vi "ExampleReader.vi"() -> ()   [LabVIEW 2011]
uses:
  Reader/readType.ctl
  2-Think/2 Typedefs/eStopCommand.ctl
  Reader/NetworkStreamReader.lvclass
panel:
  out "data 2":i32
  out "element 2":variant
  in  "Read Type":T1=enum."Most current"
  in  "Loop delay (ms)":u32
  out "element":variant
  out "data":i32
  # "Note: writer is running at 50 ms"
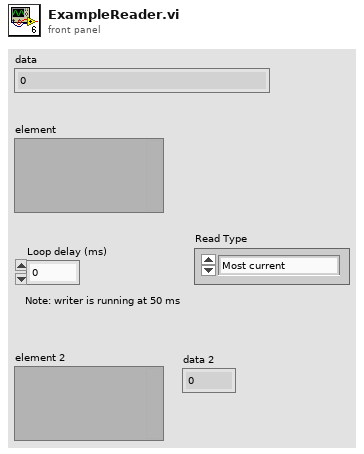
[diagram p1: front panel]
types:
  T1 = typedef "NetworkStreamReader.lvclass/readType.ctl" = enum16{"Next in buffer", "Most current"}
  T2 = typedef "eStopCommand.ctl" = enum16{"Reset E-Stop", "Get E-Stop", "Set E-Stop"}
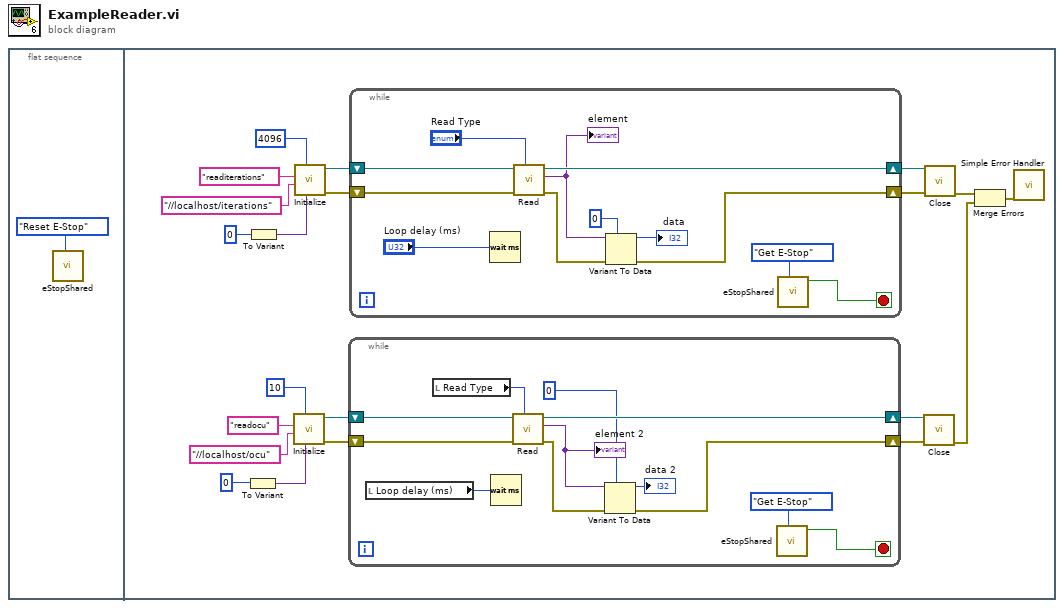
[diagram p0: block diagram]
diagram:
  n1 = flat-sequence {
    frame #0 {
      n2 = call "eStopShared.vi"("Command"=eStopCommand."Reset E-Stop") -> ()  [unwired: 9 in, 2 out]
    }
    frame #1 {
      n3 = To Variant(anything=0) -> (Variant=w13:variant)
      n4 = To Variant(anything=0) -> (Variant=w14:variant)
      n5 = call "Initialize.vi"("Default return"=w13, "writer buffer size"=10, "writer url"="//localhost/ocu", "reader name"="readocu") -> ("error out"=w6:errorcluster, "NetworkStreamWriter out"=w10:refnum<class "NetworkStreamReader.lvclass">)  [unwired: 6 in]
      n6 = call "Initialize.vi"("Default return"=w14, "writer buffer size"=4096, "writer url"="//localhost/iterations", "reader name"="readiterations") -> ("error out"=w22:errorcluster, "NetworkStreamWriter out"=w18:refnum<class "NetworkStreamReader.lvclass">)  [unwired: 6 in]
      n7 = while {
        shift-right: [w32] -> w12
        shift-left: w10 -> [w34]
        shift-right: [w23] -> w11
        shift-left: w6 -> [w33]
        stop <- w29 stop-if-true
        n8 = local read "Loop delay (ms)"() -> (w27:u32)
        n9 = local read "Read Type"() -> (w28:T1)
        n10 = Wait (ms)(milliseconds to wait=w27) -> ()  [unwired: 1 out]
        n11 = call "Read.vi"("Read Type"=w28, "error in (no error)"=w33, "NetworkStreamReader in"=w34) -> ("error out"=w24:errorcluster, "element"=w31:variant, "NetworkStreamReader out"=w32:refnum<class "NetworkStreamReader.lvclass">)  [unwired: 6 in]
        "element 2" <- w31
        n12 = Variant To Data(error in=w24, type=0, Variant=w31) -> (data=→"data 2":i32, error out=w23:errorcluster)
        n13 = call "eStopShared.vi"("Command"=eStopCommand."Get E-Stop") -> ("E-Stop Out"=w29:bool)  [unwired: 9 in, 1 out]
      }
      n14 = while {
        shift-right: [w44] -> w16
        shift-left: w18 -> [w46]
        shift-right: [w35] -> w17
        shift-left: w22 -> [w45]
        stop <- w37 stop-if-true
        n15 = Wait (ms)(milliseconds to wait="Loop delay (ms)") -> ()  [unwired: 1 out]
        n16 = call "Read.vi"("Read Type"="Read Type", "error in (no error)"=w45, "NetworkStreamReader in"=w46) -> ("error out"=w36:errorcluster, "element"=w43:variant, "NetworkStreamReader out"=w44:refnum<class "NetworkStreamReader.lvclass">)  [unwired: 6 in]
        "element" <- w43
        n17 = Variant To Data(error in=w36, type=0, Variant=w43) -> (data=→"data":i32, error out=w35:errorcluster)
        n18 = call "eStopShared.vi"("Command"=eStopCommand."Get E-Stop") -> ("E-Stop Out"=w37:bool)  [unwired: 9 in, 1 out]
      }
      n19 = call "Close.vi"("error in (no error)"=w11, "NetworkStreamReader in"=w12) -> ("error out"=w4:errorcluster)  [unwired: 8 in, 1 out]
      n20 = call "Close.vi"("error in (no error)"=w17, "NetworkStreamReader in"=w16) -> ("error out"=w5:errorcluster)  [unwired: 8 in, 1 out]
      n21 = Merge Errors(w5, w4) -> (w3:errorcluster)
      n22 = call <vilib>:"Simple Error Handler.vi"("error in (no error)"=w3) -> ()  [unwired: 4 in, 5 out]
    }
  }
